vi "KE6221 -- Set Wave Phase Marker.vi"(0 "Resource In":refnum<visa-resource-name>, 1 "Check For SCPI Errors? (T)":bool=TRUE, 7 "Phase Marker In (deg)":T1=180.0 min=0.0 max=360.0 format="%.3f", 11 "error in (no error)":errorcluster, 12 "Read Back Set Value? (T)":bool=TRUE) -> (4 "Resource Out (dupl)":refnum<visa-resource-name>, 8 "Phase Marker Out (deg)":T1=180.0 min=0.0 max=360.0 format="%.3f", 15 "error out":errorcluster)   [LabVIEW 2018, in "Keithley 622x.lvlib"]
uses:
  Keithley 622x.lvlib
  Typedefs/KE6221 -- Wave Phase Marker.ctl
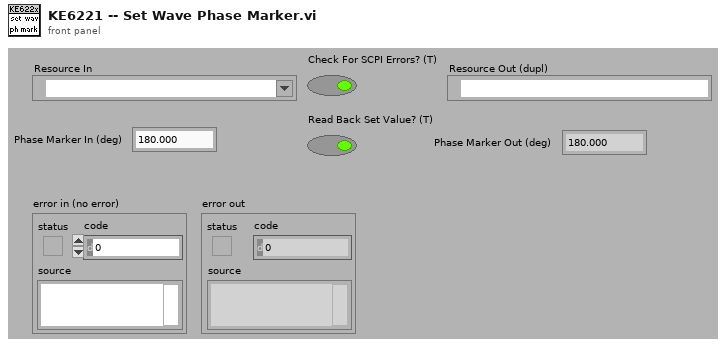
[diagram p1: front panel]
types:
  T1 = typedef "Keithley 622x.lvlib/KE6221 -- Wave Phase Marker.ctl" = dbl
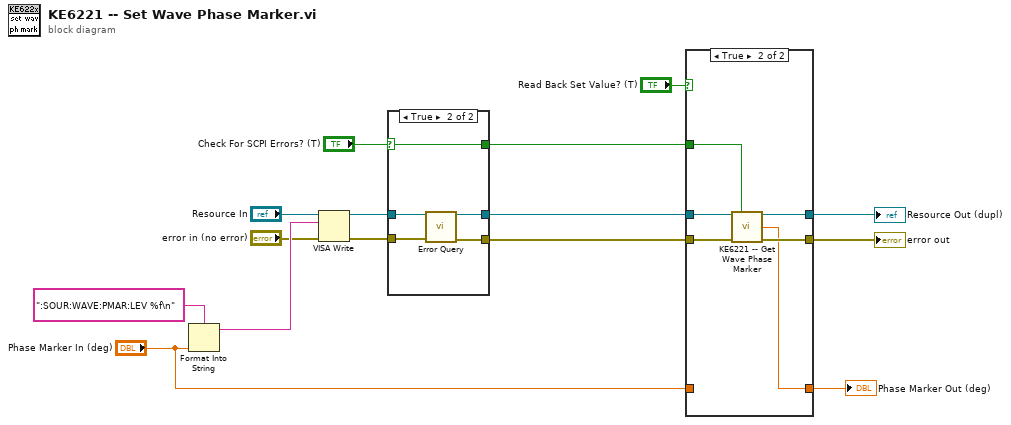
[diagram p0: block diagram]
diagram:
  n1 = Format Into String(format string=":SOUR:WAVE:PMAR:LEV %f\n", "Phase Marker In (deg)") -> (resulting string=w13:string)  [unwired: 2 in, 1 out]
  n2 = VISA Write(VISA resource name="Resource In", write buffer=w13, error in (no error)="error in (no error)") -> (VISA resource name out=w10:refnum<visa-resource-name>, error out=w9:errorcluster)  [unwired: 1 out]
  n3 = case shown="True" "Check For SCPI Errors? (T)" {
    selector: "Check For SCPI Errors? (T)" -> [w16 w19]
    tunnel: w10 -> [w18 w23]
    tunnel: w9 -> [w17 w22]
    tunnel: [w17 w21] -> w5
    tunnel: [w18 w20] -> w8
    tunnel: [w16 w19] -> w6
    frame False {
    }
    frame True {
      n4 = call "Error Query.vi"("VISA Resource In"=w23, "error in (no error)"=w22) -> ("VISA Resource Out (dupl)"=w20:refnum<visa-resource-name>, "error out"=w21:errorcluster)  [unwired: 10 in, 2 out]
    }
  }
  n5 = case shown="True" "Read Back Set Value? (T)" {
    tunnel: w8 -> [w25 w32]
    tunnel: w6 -> [_ w31]
    tunnel: w5 -> [w24 w30]
    tunnel: "Phase Marker In (deg)" -> [w26 _]
    tunnel: [w26 w27] -> w1
    tunnel: [w25 w29] -> w4
    tunnel: [w24 w28] -> w3
    frame False {
    }
    frame True {
      n6 = call "KE6221 -- Get Wave Phase Marker.vi"("Resource In"=w32, "Check For SCPI Errors? (T)"=w31, "error in (no error)"=w30) -> ("Resource Out (dupl)"=w29:refnum<visa-resource-name>, "Phase Marker (deg)"=w27:T1, "error out"=w28:errorcluster)  [unwired: 10 in]
    }
  }
  "Resource Out (dupl)" <- w4
  "error out" <- w3
  "Phase Marker Out (deg)" <- w1
